vi "getSpectrum.vi"(8 "error in (no error)":errorcluster, 11 "Model in":refnum<class "Model.lvclass">) -> (0 "error out":errorcluster, 1 "intensity[2048]":dbl[](array[numeric]), 2 "wavelength[2048]":dbl[](array[numeric]), 3 "Model out":refnum<class "Model.lvclass">)   [LabVIEW 2016, in "Model.lvclass"]
uses:
  Model.lvclass
  Model.lvclass/Model.ctl
  ss_sedspectrometer/SEDSpectrometer/SEDSpectrometer.lvclass
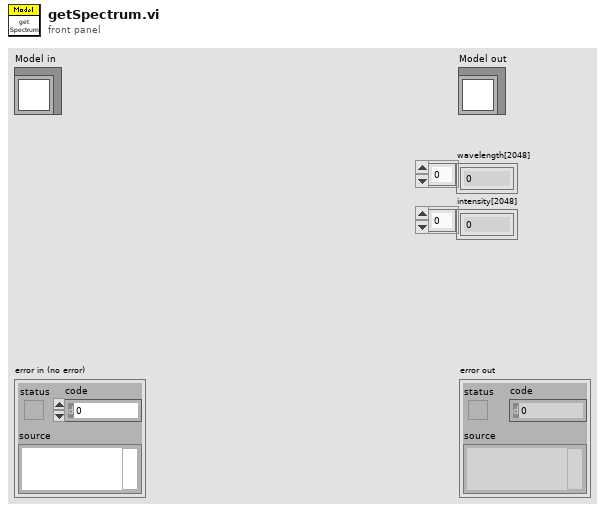
[diagram p1: front panel]
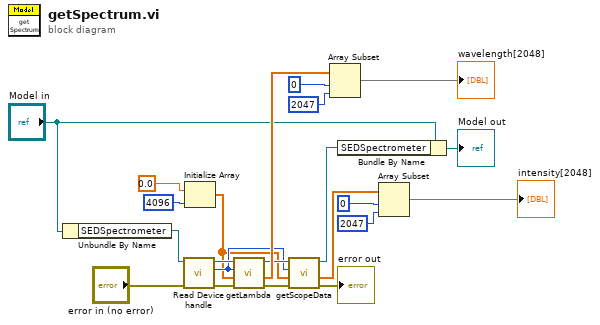
[diagram p0: block diagram]
diagram:
  n1 = Unbundle By Name("Model in") -> ("SEDSpectrometer"=w22:refnum<class "SEDSpectrometer.lvclass">)
  n2 = call-dynamic "Read Device handle.vi"("error in (no error)"="error in (no error)", "SEDSpectrometer in"=w22) -> ("error out"=w1:errorcluster, "Device handle"=w12:i32, "SEDSpectrometer out"=w20:refnum<class "SEDSpectrometer.lvclass">)  [unwired: 7 in]
  n3 = Initialize Array(0.0, 4096 ("dimension size")) -> (w11:dbl[])
  n4 = call "getLambda.vi"("error in (no error)"=w1, "WaveLength In"=w11, "Device"=w12, "SEDSpectrometer in"=w20) -> ("error out"=w2:errorcluster, "WaveLength Out"=w15:dbl[], "SEDSpectrometer out"=w13:refnum<class "SEDSpectrometer.lvclass">)  [unwired: 4 in, 1 out]
  n5 = call "getScopeData.vi"("error in (no error)"=w2, "Spectrum"=w11, "Device"=w12, "SEDSpectrometer in"=w13) -> ("error out"=→"error out":errorcluster, "Spectrum"=w8:dbl[], "SEDSpectrometer out"=w7:refnum<class "SEDSpectrometer.lvclass">)  [unwired: 4 in, 1 out]
  n6 = Array Subset(array=w15, index=0, length=2047) -> (→"wavelength[2048]":dbl[])
  n7 = Bundle By Name(cluster="Model in", "SEDSpectrometer"=w7) -> (→"Model out":refnum<class "Model.lvclass">)
  n8 = Array Subset(array=w8, index=0, length=2047) -> (→"intensity[2048]":dbl[])
